vi "GET.vi"(6 "timeout":i32=10000, 7 "output file":path, 8 "error in":errorcluster, 10 "url":string, 11 "advanced-http-client in":refnum<class "advanced-http-client.lvclass">) -> (0 "error out":errorcluster, 2 "response":refnum<class "response.lvclass">, 3 "advanced-http-client out":refnum<class "advanced-http-client.lvclass">)   [LabVIEW 2020, in "advanced-http-client.lvclass"]
uses:
  advanced-http-client.lvclass
  advanced-http-client.lvclass/advanced-http-client.ctl
  <vilib>/NI/Advanced HTTP Client/Session.lvclass
  response/response.lvclass
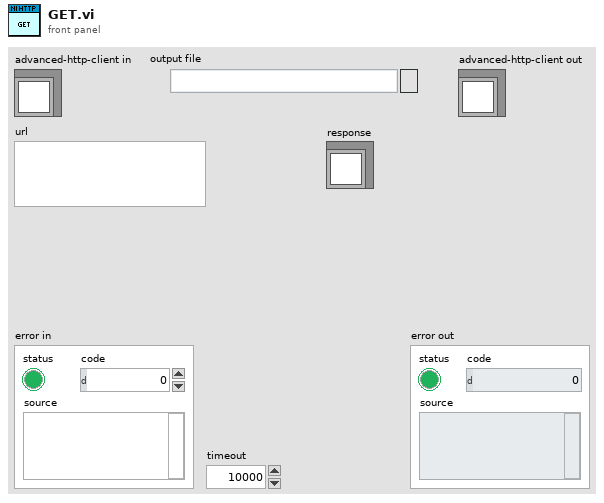
[diagram p1: front panel]
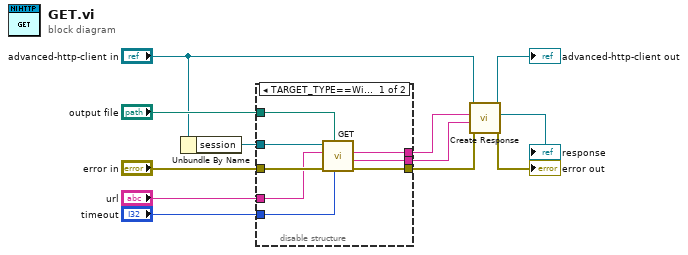
[diagram p0: block diagram]
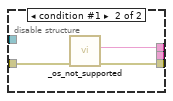
[diagram p2: hidden frame]
diagram:
  n1 = Unbundle By Name("advanced-http-client in") -> ("session"=w12:refnum<class "Session.lvclass">)
  n2 = disable-structure shown="TARGET_TYPE==Windows" {
    disable-tunnel: w12 -> [w20 _]
    disable-tunnel: "output file" -> [w19 _]
    disable-tunnel: "error in" -> [w18 w23]
    disable-tunnel: [w17 w22] -> w4
    disable-tunnel: [w16 w21] -> w2
    disable-tunnel: "timeout" -> [w15 _]
    disable-tunnel: "url" -> [w14 _]
    disable-tunnel: [w13 _] -> w5
    frame condition #0 (active) {
      n3 = call <vilib>:"GET.vi"("timeout"=w15, "output file"=w19, "error in"=w18, "url"=w14, "session in"=w20) -> ("error out"=w17:errorcluster, "body"=w13:string, "headers"=w16:string)  [unwired: 2 in, 2 out]
    }
    frame condition #1 {
      n4 = call "_os_not_supported.vi"("error in (no error)"=w23) -> ("error out"=w22:errorcluster, "headers"=w21:string)  [unwired: 9 in]
    }
  }
  n5 = call-dynamic "Create Response.vi"("error in (no error)"=w4, "body"=w5, "headers"=w2, "http-client"="advanced-http-client in") -> ("error out"=→"error out":errorcluster, "response out"=→"response":refnum<class "response.lvclass">, "http-client out"=→"advanced-http-client out":refnum<class "advanced-http-client.lvclass">)  [unwired: 5 in]
